vi "LoadControlPanel.vi"(8 "error in (no error)":errorcluster, 10 "Actor In":refnum<class "Actor.lvclass">, 11 "Stage_MadCityLab in":refnum<class "Stage_MadCityLab.lvclass">) -> (0 "error out":errorcluster, 3 "Stage_MadCityLab out":refnum<class "Stage_MadCityLab.lvclass">)   [LabVIEW 2020, in "Stage_MadCityLab.lvlib" / "Stage_MadCityLab.lvclass"]
uses:
  Stage_MadCityLab.lvclass
  <vilib>/ActorFramework/Actor/Actor.lvclass
  ViewController/TripleAxisStageController/TriaxesStageController.lvclass
  C:/Program Files/National Instruments/LabVIEW 2020/vi.lib/ActorFramework/Actor/Actor.lvclass
  Hardware Abstraction Layer/Component/Stage/Stage/Stage.lvclass
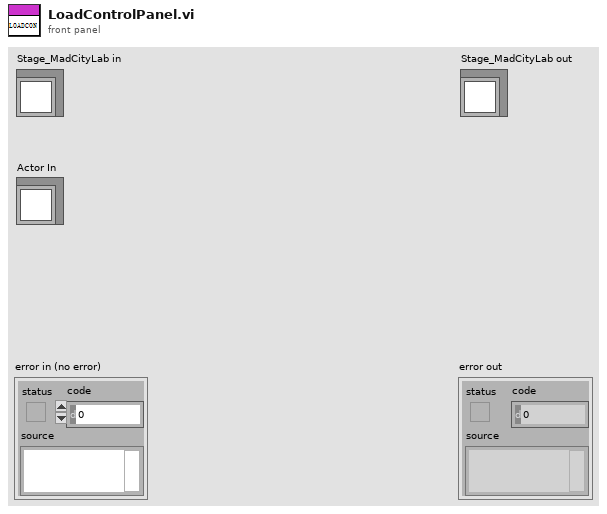
[diagram p1: front panel]
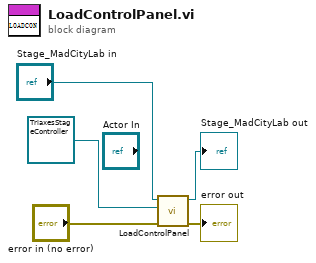
[diagram p0: block diagram]
diagram:
  n1 = call-parent "LoadControlPanel.vi"("error in (no error)"="error in (no error)", "Actor In"=refnum<class "TriaxesStageController.lvclass"> refnum ("TripleAxisStageController.lvlib:TripleAxisStageController.lvclass"), "GRMActor in"="Stage_MadCityLab in") -> ("error out"=→"error out":errorcluster, "GRMActor out"=→"Stage_MadCityLab out":refnum<class "Stage_MadCityLab.lvclass">)  [unwired: 7 in]
